vi "Gen_Test_Single_Cell.vi"() -> ()   [LabVIEW 2020]
uses:
  Battery-Testing-Software-NHR/system_development/v0.1/Drivers-NHR-9200/NHR/NH Research Regenerative Test Series.lvlib
panel:
  in  "Charge time":dbl
  in  "Discharge time":dbl
  in  "Data Task in 2":refnum<k21>
  in  "Output Safety":T1
  in  "filepath":path
  in  "Batteryname":string
  in  "Starting Cycle":i32
  out "PS error out":errorcluster
  out "data task error out":errorcluster
  out "data task out":refnum<k21>
  in  "Charge Current Cutoff":dbl
  in  "Charge Current Setpoint 2":dbl format="%#.6g"
  in  "charge Voltage Setpoint  2":dbl format="%#.6g"
  in  "Wait time":dbl
  in  "Discharge Current Cutoff":dbl
  in  "Discharge Current Setpoint":dbl format="%#.6g"
  in  "Discharge Voltage Setpoint":dbl format="%#.6g"
  in  "data task error in":errorcluster
  in  "NHR VISA":refnum<visa-resource-name>
  in  "NHR error in":errorcluster
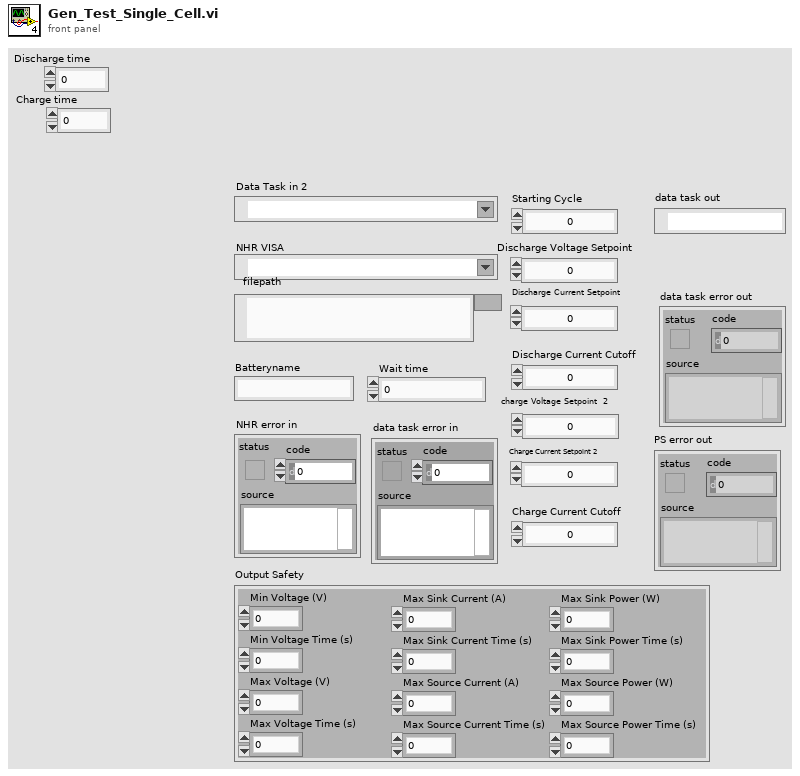
[diagram p1: front panel]
types:
  T1 = cluster{"Min Voltage (V)":dbl, "Min Voltage Time (s)":dbl, "Max Voltage (V)":dbl, "Max Voltage Time (s)":dbl, "Max Sink Current (A)":dbl, "Max Sink Current Time (s)":dbl, "Max Source Current (A)":dbl, "Max Source Current Time (s)":dbl, "Max Sink Power (W)":dbl, "Max Sink Power Time (s)":dbl, "Max Source Power (W)":dbl, "Max Source Power Time (s)":dbl}
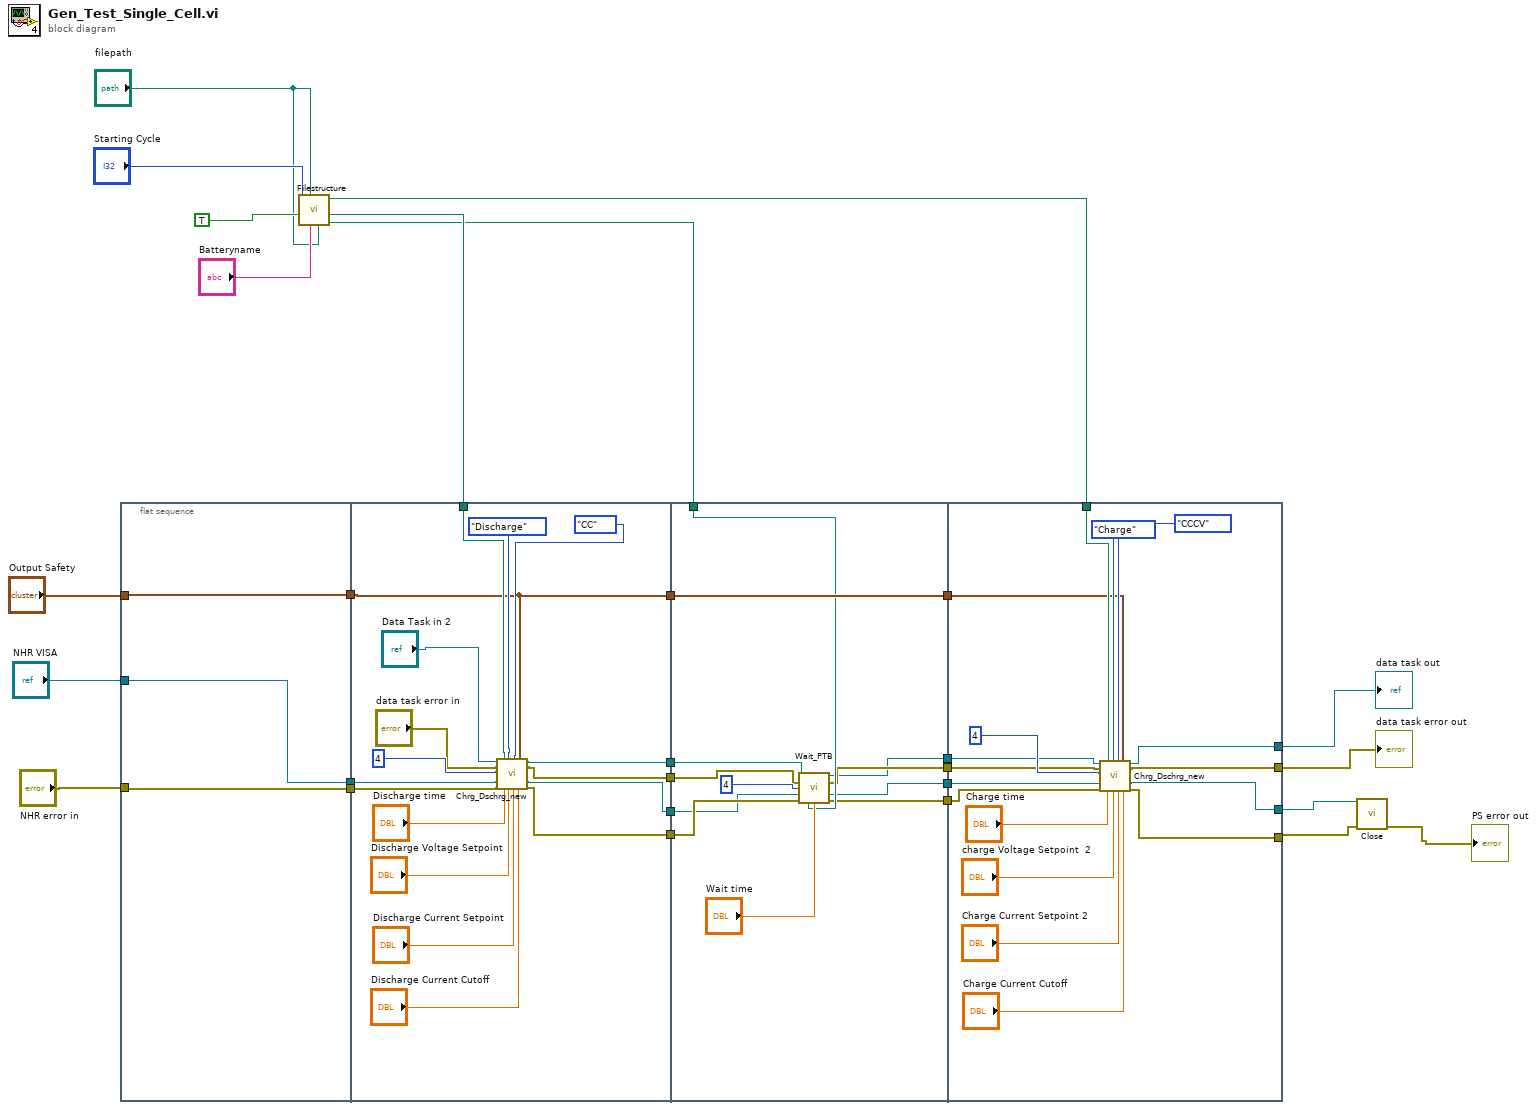
[diagram p0: block diagram]
diagram:
  n1 = flat-sequence {
    tunnel: "NHR error in" -> [w30]
    tunnel: "NHR VISA" -> [w31]
    tunnel: [w31] -> w26
    tunnel: [w30] -> w25
    tunnel: "Output Safety" -> [w29]
    tunnel: [w29] -> w12
    tunnel: w26 -> [w40]
    tunnel: w25 -> [w41]
    tunnel: [w48] -> w24
    tunnel: [w47] -> w23
    tunnel: [w46] -> w22
    tunnel: [w45] -> w21
    tunnel: w15 -> [w37]
    tunnel: w12 -> [w34]
    tunnel: [w34] -> w11
    tunnel: w24 -> [w56]
    tunnel: w23 -> [w57]
    tunnel: w22 -> [w49]
    tunnel: w21 -> [w59]
    tunnel: w14 -> [w54]
    tunnel: w11 -> [w60]
    tunnel: [w60] -> w10
    tunnel: [w53] -> w7
    tunnel: [w52] -> w6
    tunnel: [w51] -> w5
    tunnel: [w50] -> w4
    tunnel: [w69] -> w2
    tunnel: [w68] -> w3
    tunnel: [w66] -> w20
    tunnel: [w67] -> w19
    tunnel: w13 -> [w73]
    tunnel: w10 -> [w70]
    tunnel: w7 -> [w65]
    tunnel: w6 -> [w64]
    tunnel: w5 -> [w63]
    tunnel: w4 -> [w62]
    frame #0 {
    }
    frame #1 {
      n2 = call "Chrg_Dschrg_new.vi"("Data Task in"="Data Task in 2", "data task error in"="data task error in", "#DAQ outputs (1-13)"=4, "PS VISA in"=w40, "PS error in"=w41, "DischargeCyclePath"=w37, "Charge/Discharge\n time"="Discharge time", "Charge/discharge"=enum8{"Charge", "Discharge"}."Discharge", "Charge/Discharge Voltage Setpoint"="Discharge Voltage Setpoint", "CC or CCCV"=enum16{"CC", "CCCV"}."CC", "Current Setpoint"="Discharge Current Setpoint", "Output Safety"=w34, "Current Cutoff"="Discharge Current Cutoff") -> ("data task out"=w48:refnum<k21>, "data task error out"=w47:errorcluster, "PS VIS resource name out"=w46:refnum<visa-resource-name>, "PS error out"=w45:errorcluster)  [unwired: 3 in]
    }
    frame #2 {
      n3 = call "Wait_PTB.vi"("Data Task in"=w56, "data task error in"=w57, "#DAQ outputs (1-13)"=4, "PS VISA in"=w49, "PS error in"=w59, "Wait Filepath"=w54, "Wait time"="Wait time") -> ("data task out"=w50:refnum<k21>, "data task error out"=w51:errorcluster, "PS Visa Out"=w52:refnum<visa-resource-name>, "PS error out"=w53:errorcluster)  [unwired: 5 in]
    }
    frame #3 {
      n4 = call "Chrg_Dschrg_new.vi"("Data Task in"=w62, "data task error in"=w63, "#DAQ outputs (1-13)"=4, "PS VISA in"=w64, "PS error in"=w65, "DischargeCyclePath"=w73, "Charge/Discharge\n time"="Charge time", "Charge/discharge"=enum8{"Charge", "Discharge"}."Charge", "Charge/Discharge Voltage Setpoint"="charge Voltage Setpoint  2", "CC or CCCV"=enum16{"CC", "CCCV"}."CCCV", "Current Setpoint"="Charge Current Setpoint 2", "Output Safety"=w70, "Current Cutoff"="Charge Current Cutoff") -> ("data task out"=w66:refnum<k21>, "data task error out"=w67:errorcluster, "PS VIS resource name out"=w68:refnum<visa-resource-name>, "PS error out"=w69:errorcluster)  [unwired: 3 in]
    }
  }
  n5 = call "Filestructure.vi"("Discharge filepath"="filepath", "Batteryname"="Batteryname", "Charge filepath"="filepath", "In for loop"=TRUE, "Starting Cycle"="Starting Cycle") -> ("DischargeWaitPath"=w14:path, "DischargeCyclePath"=w15:path, "ChargeCyclePath"=w13:path)  [unwired: 2 in, 2 out]
  n6 = call "Close.vi"("VISA resource name"=w3, "error in (no error)"=w2) -> ("error out"=→"PS error out":errorcluster)  [unwired: 13 in]
  "data task out" <- w20
  "data task error out" <- w19
